vi "Execute Multiple Commands with a Single Channel.vi"() -> ()   [LabVIEW 2018]
doc: "Executes multiple commands using a single channel to a remote SSH server. This is similar to logging into a remote SSH server through a terminal, executing multiple commands at the prompt, and then logging out of the remote SSH server. For a more interactive experience, like a Read-Evaluate-Print-Loop (REPL), a while loop and some more complexity would be required."
uses:
  Toolkit/Channel/Channel.lvclass/Channel.ctl
  Toolkit/Session/Session.lvclass/Session.ctl
  Toolkit/SSH/SSH.lvclass/SSH.ctl
  Toolkit/Session/Utility/Read Shared Library.vi
  Toolkit/SSH/Utility/Read Shared Library.vi
  Toolkit/Session/Support/Create from SSH.vi
  Toolkit/Session/Support/Password Authentication.vi
  Toolkit/Channel/Support/Create from Session.vi
  Toolkit/Support/Check Status.vi
  Toolkit/Channel/Support/Destroy to Session.vi
  Toolkit/Session/Support/Destroy to SSH.vi
  Toolkit/SSH/SSH.lvclass
  Toolkit/Session/Session.lvclass
  Toolkit/Channel/Channel.lvclass
panel:
  out "Login Message Size":i32 caption="Login Size"
  in  "Max Login Message Size":u64=1024 caption="Max Login Size"
  out "Response 2 Size":i32 caption="Response Size"
  in  "Command 2 Max Response Size":u64=1024 caption="Max Response Size"
  out "Response 1 Size":i32 caption="Response Size"
  in  "Command 1 Max Response Size":u64=1024 caption="Max Response Size"
  in  "Timeout":i32=500 caption="Timeout (ms)"
  out "Login Message":string
  out "Response 2":string
  in  "Command 2":string="echo \"Hello World from the second command!\""
  out "Response 1":string
  in  "Command 1":string="echo \"Hello World from the first command!\""
  in  "Address":string
  in  "Password":string
  in  "Username":string
  # "Overview: Demonstrates executing a multiple, sequential commands using a single Shell channel\nInstructions:\n1. Enter the IP address or host name of the remote SSH server. This can be a CompactRIO (cRIO) running the National instruments Linux Real-Time (NI Linux RT) operating system with the Enable Secure Shell Server (sshd) checkbox checked.\n2. Enter a username. If using a cRIO with a default configuration, then the username is \"admin\".\n3. Enter the password for the username. If using a cRIO with a default configuration, then the password is blank (empty).\n4. Run this VI.\n5. Observe the login message. Some remote SSH servers may not display a login message.\n6. Observe \"Hello World from the first command!\" and \"Hello World from the second command!\" for Response 1 and 2, respectively.\n7. Change Command 1 and Command 2.\n8. Rerun this VI.\n9. Observe the responses for Command 1 and Command 2, respectively."
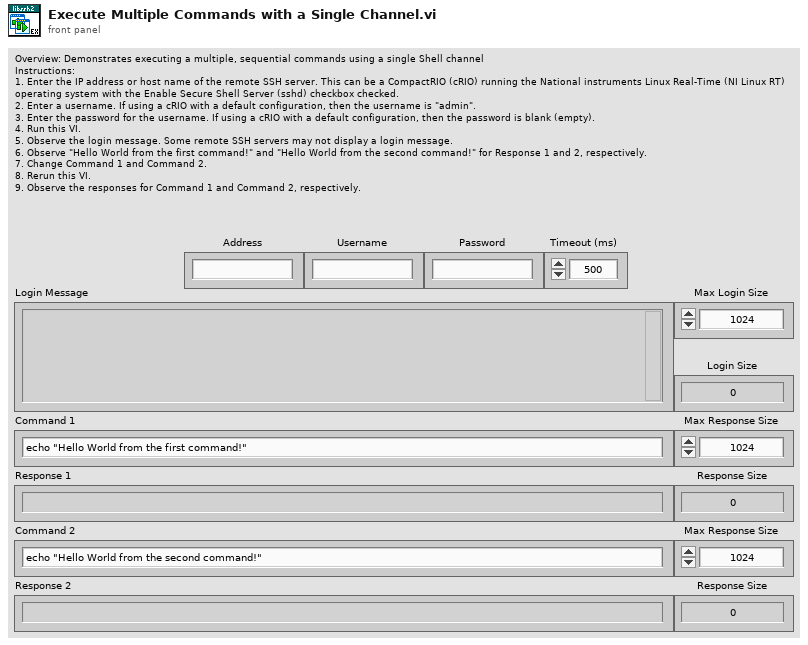
[diagram p1: front panel]
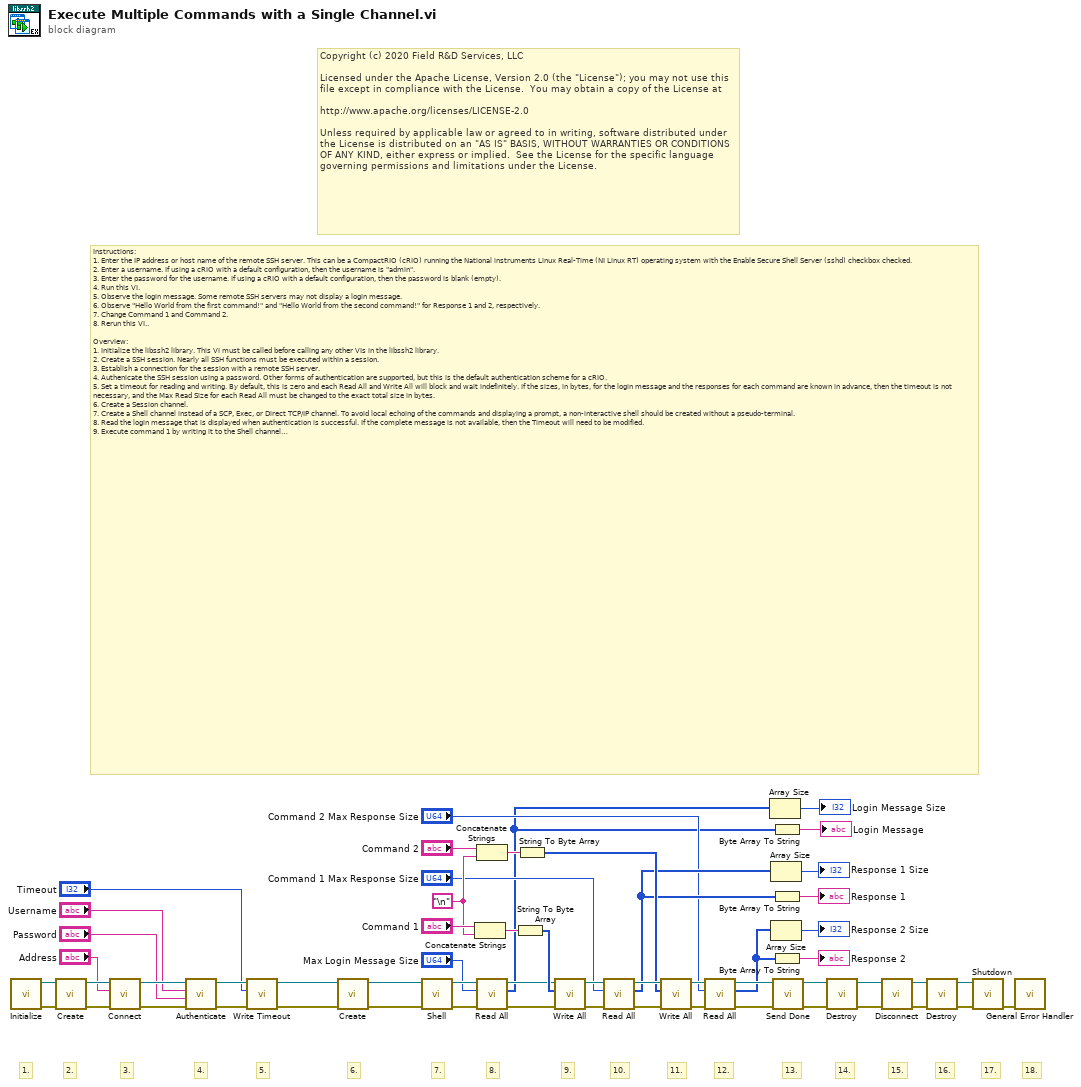
[diagram p0: block diagram]
diagram:
  w22 = "\n"
  # "18."
  # "Copyright (c) 2020 Field R&D Services, LLC\n\nLicensed under the Apache License, Version 2.0 (the \"License\"); you may not use this file except in compliance with the License.  You may obtain a copy of the License at\n\nhttp://www.apache.org/licenses/LICENSE-2.0\n\nUnless required by applicable law or agreed to in writing, software distributed under the License is distributed on an \"AS IS\" BASIS, WITHOUT WARRANTIES OR CONDITIONS OF ANY KIND, either express or implied.  See the License for the specific language governing permissions and limitations under the License."
  # "17."
  # "16."
  # "15."
  # "14."
  # "13."
  # "12."
  # "11."
  # "10."
  # "9."
  # "8."
  # "7."
  # "6."
  # "5."
  # "4."
  # "3."
  # "2."
  # "1."
  # "Instructions:\n1. Enter the IP address or host name of the remote SSH server. This can be a CompactRIO (cRIO) running the National instruments Linux Real-Time (NI Linux RT) operating system with the Enable Secure Shell Server (sshd) checkbox checked.\n2. Enter a username. If using a cRIO with a default configuration, then the username is \"admin\".\n3. Enter the password for the username. If using a cRIO with a default configuration, then the password is blank (empty).\n4. Run this VI.\n5. Observe the login message. Some remote SSH servers may not display a login message.\n6. Observe \"Hello World from the first command!\" and \"Hello World from the second command!\" for Response 1 and 2, respectively.\n7. Change Command 1 and Command 2.\n8. Rerun this VI..\n\nOverview:\n1. Initialize the libssh2 library. This VI must be called before calling any other VIs in the libssh2 library.\n2. Create a SSH session. Nearly all SSH functions must be executed within a session.\n3. Establish a connection for the session with a remote SSH server.\n4. Authenicate the SSH session using a password. Other forms of authentication are supported, but this is the default authentication scheme for a cRIO. \n5. Set a timeout for reading and writing. By default, this is zero and each Read All and Write All will block and wait indefinitely. If the sizes, in bytes, for the login message and the responses for each command are known in advance, then the timeout is not necessary, and the Max Read Size for each Read All must be changed to the exact total size in bytes.\n6. Create a Session channel.\n7. Create a Shell channel instead of a SCP, Exec, or Direct TCP/IP channel. To avoid local echoing of the commands and displaying a prompt, a non-interactive shell should be created without a pseudo-terminal.\n8. Read the login message that is displayed when authentication is successful. If the complete message is not available, then the Timeout will need to be modified.\n9. Execute command 1 by writing it to the Shell channel. The Command 1 Max Response Size is the maximum response size in bytes (B) from the output of executing Command 1. If Timeout is zero (0), then this value must be the exact number of bytes to avoid stalling and waiting indefinitely.\n10. Read the first response. If Timeout is zero (0), then this value will match the Command 1 Max Response Size value.\n11. Execute command 2 by writing it to the Shell channel. The Command 2 Max Response Size is the maximum response size in bytes (B) from the output of executing Command 2. If Timeout is zero (0), then this value must be the exact number of bytes to avoid stalling and waiting indefinitely.\n12. Read the second response. If Timeout is zero (0), then this value will match the Command 1 Max Response Size value.\n13. Signal completion of the Session channel to the remote server. Not strictly required, but it is good practice. \n14. Destroy the Session channel. Since the \"Create\" VI is used, the complementary \"Destroy\" VI must be used to free resources within the libssh2 library. \n15. Disconnect from the remote SSH server.\n16. Destroy the session to free resources within the libssh2 library.\n17. Shutdown the libssh2 library. This VI must be last VI called for the libssh2 library. No other libssh2 VIs should be called once this VI is executed.\n18. Provide some error handling and reporting. Libssh2 errors will be in the -8100 range while warnings will be in the 5000 range."
  n1 = call "Initialize.vi"() -> ("Error Out"=w55:errorcluster, "SSH"=w56:refnum<class "SSH.lvclass">)  [unwired: 10 in]
  n2 = call-poly "Create.vi"("Error In"=w55, "SSH"=w56) -> ("Error Out"=w53:errorcluster, "Sesssion"=w54:refnum<class "Session.lvclass">)  [unwired: 8 in]
  n3 = call "Connect.vi"("Error In"=w53, "Address"="Address", "Session In"=w54) -> ("Error Out"=w51:errorcluster, "Sesssion Out"=w52:refnum<class "Session.lvclass">)  [unwired: 7 in]
  n4 = call-poly "Authenticate.vi"("Error In"=w51, "Password"="Password", "Username"="Username", "Session In"=w52) -> ("Error Out"=w14:errorcluster, "Sesssion Out"=w15:refnum<class "Session.lvclass">)  [unwired: 6 in]
  n5 = call "Write Timeout.vi"("Error In"=w14, "Timeout"="Timeout", "Session In"=w15) -> ("Error Out"=w13:errorcluster, "Sesssion Out"=w12:refnum<class "Session.lvclass">)  [unwired: 7 in]
  n6 = call-poly "Create.vi"("Error In"=w13, "Session"=w12) -> ("Error Out"=w20:errorcluster, "Channel"=w21:refnum<class "Channel.lvclass">)  [unwired: 8 in]
  n7 = call "Shell.vi"("Error In"=w20, "Channel In"=w21) -> ("Error Out"=w18:errorcluster, "Channel Out"=w19:refnum<class "Channel.lvclass">)  [unwired: 8 in]
  n8 = Concatenate Strings("Command 1", w22) -> (w25:string)
  n9 = Concatenate Strings("Command 2", w22) -> (w23:string)
  n10 = call "Read All.vi"("Error In"=w18, "Max Read Size"="Max Login Message Size", "Channel In"=w19) -> ("Error Out"=w11:errorcluster, "Data"=w2:u8[], "Channel Out"=w27:refnum<class "Channel.lvclass">)  [unwired: 5 in, 1 out]
  n11 = String To Byte Array(string=w25) -> (unsigned byte array=w36:u8[])
  n12 = String To Byte Array(string=w23) -> (unsigned byte array=w28:u8[])
  n13 = call "Write All.vi"("Error In"=w11, "Data"=w36, "Channel In"=w27) -> ("Error Out"=w17:errorcluster, "Channel Out"=w35:refnum<class "Channel.lvclass">)  [unwired: 5 in, 2 out]
  n14 = call "Read All.vi"("Error In"=w17, "Max Read Size"="Command 1 Max Response Size", "Channel In"=w35) -> ("Error Out"=w33:errorcluster, "Data"=w9:u8[], "Channel Out"=w34:refnum<class "Channel.lvclass">)  [unwired: 5 in, 1 out]
  n15 = call "Write All.vi"("Error In"=w33, "Data"=w28, "Channel In"=w34) -> ("Error Out"=w31:errorcluster, "Channel Out"=w32:refnum<class "Channel.lvclass">)  [unwired: 5 in, 2 out]
  n16 = call "Read All.vi"("Error In"=w31, "Max Read Size"="Command 2 Max Response Size", "Channel In"=w32) -> ("Error Out"=w30:errorcluster, "Data"=w5:u8[], "Channel Out"=w29:refnum<class "Channel.lvclass">)  [unwired: 5 in, 1 out]
  n17 = Array Size(array=w2) -> (size(s)=→"Login Message Size":i32)
  n18 = Array Size(array=w9) -> (size(s)=→"Response 1 Size":i32)
  n19 = Array Size(array=w5) -> (size(s)=→"Response 2 Size":i32)
  n20 = Byte Array To String(unsigned byte array=w2) -> (string=→"Login Message":string)
  n21 = Byte Array To String(unsigned byte array=w9) -> (string=→"Response 1":string)
  n22 = Byte Array To String(unsigned byte array=w5) -> (string=→"Response 2":string)
  n23 = call "Send Done.vi"("Error In"=w30, "Channel In"=w29) -> ("Error Out"=w49:errorcluster, "Channel Out"=w50:refnum<class "Channel.lvclass">)  [unwired: 8 in]
  n24 = call-poly "Destroy.vi"("Error In"=w49, "Channel"=w50) -> ("Error Out"=w47:errorcluster, "Session"=w48:refnum<class "Session.lvclass">)  [unwired: 8 in]
  n25 = call "Disconnect.vi"("Error In"=w47, "Session In"=w48) -> ("Error Out"=w45:errorcluster, "Sesssion Out"=w46:refnum<class "Session.lvclass">)  [unwired: 8 in]
  n26 = call-poly "Destroy.vi"("Error In"=w45, "Session"=w46) -> ("Error Out"=w43:errorcluster, "SSH"=w44:refnum<class "SSH.lvclass">)  [unwired: 8 in]
  n27 = call "Shutdown.vi"("Error In"=w43, "SSH"=w44) -> ("Error Out"=w38:errorcluster)  [unwired: 9 in]
  n28 = call <vilib>:"General Error Handler.vi"("error in (no error)"=w38) -> ()  [unwired: 10 in, 5 out]
